vi "AMZ_S3_APIHLP_Convert StorageClass String to Enum.vi"(4 "Storage Class String":string) -> (1 "Storage Class":T1)   [LabVIEW 2015, in "LV Interface for Amazon S3.lvlib"]
doc: "Convert the Storage Class represented as a String to the Enum typedef representation."
uses:
  LV Interface for Amazon S3.lvlib
  Typedefs/AMZ_S3_Storage Class.ctl
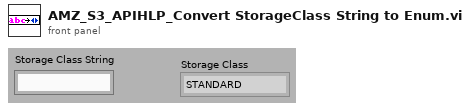
[diagram p1: front panel]
types:
  T1 = typedef "LV Interface for Amazon S3.lvlib/AMZ_S3_Storage Class.ctl" = enum16{"STANDARD", "REDUCED_REDUNDANCY"}
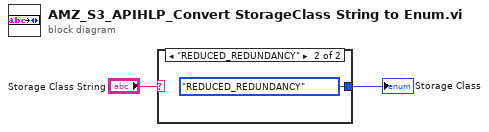
[diagram p0: block diagram]
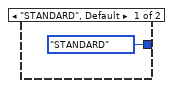
[diagram p2: hidden frame]
diagram:
  n1 = case shown="\"REDUCED_REDUNDANCY\"" "Storage Class String" {
    tunnel: [AMZ_S3_Storage_Class."STANDARD" ("Storage Class") AMZ_S3_Storage_Class."REDUCED_REDUNDANCY" ("Storage Class")] -> w1
    frame "STANDARD", Default {
    }
    frame "REDUCED_REDUNDANCY" {
    }
  }
  "Storage Class" <- w1
